vi "Drive Teleop Handler.vi"(10 "Call Context":T1) -> ()   [LabVIEW 2023]
uses:
  swerve/Type Definitions/Data/Robot Velocities.ctl
  <vilib>/Rock Robotics/WPI/DriverStation/WPI_DriverStationDerivedRobotMode.ctl
  Drive/Implementation/Driving Mode.ctl
  <vilib>/Rock Robotics/WPI/Joystick/XBox Buttons Indexer.ctl
  ce51abe2-3967-49ec-91df-d4b8ef358bb3.vi
  20f039dc-a6f5-4e97-88ba-31848a91c715.vi
  2558f998-dd4e-4154-8f44-6f70b21d0474.vi
  fdc21bd4-9215-41b8-8367-bf19dde4ba27.vi
  <vilib>/Rock Robotics/WPI/Utilities/WPI_GetSetVariantRefNum.vi
  <vilib>/Rock Robotics/Network Tables/NT Read Number.vi
  <vilib>/Rock Robotics/Network Tables/NT Read Boolean.vi
  <vilib>/Rock Robotics/Network Tables/NT Write Boolean.vi
  Framework/Robot Global Data.vi
panel:
  in  "Deadband Info":T2={"Deadband"=0.05, "Deadband High"=1.0, "Deadband Low"=0.05}
  in  "Max Velocities":T3={"X Velocity"=15.0, "Y Velocity"=15.0, "Rotational \nVelocity"=270.0}
  in  "Sinusoidal Terms":cluster{"Max Velocity":dbl, "Frequency":dbl}
  in  "Teleop Mode":T4(ring)
  in  "Joystick Inputs":T5(array[cluster])
  in  "Send Inputs":bool
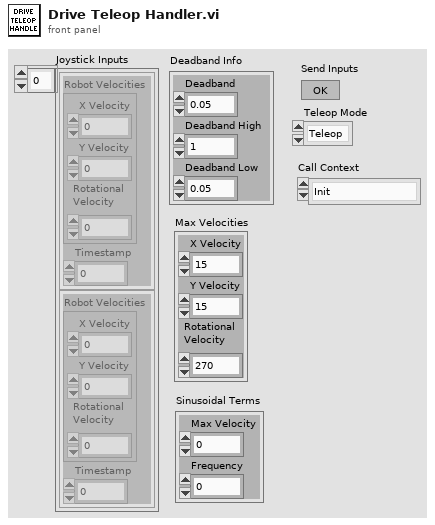
[diagram p1: front panel]
types:
  T1 = typedef "WPI_DriverStationDerivedRobotMode.ctl" = enum16{"Init", "Execute", "Stop"}
  T2 = cluster{"Deadband":dbl, "Deadband High":dbl, "Deadband Low":dbl}
  T3 = typedef "Robot Velocities.ctl" = cluster{"X Velocity":dbl, "Y Velocity":dbl, "Rotational \nVelocity":dbl}
  T4 = enum16{"Teleop", "Simulated Teleop", "Sine Velocity Profiles", "Circle Simulator"}
  T5 = cluster{"Robot Velocities":T3, "Timestamp":dbl}[]
  T6 = typedef "XBox Buttons Indexer.ctl" = enum16{"A", "B", "X", "Y", "Left Bumper", "Right Bumper", "Back", "Start", "Left Joystick", "Right Joystick"}
  T7 = typedef "Driving Mode.ctl" = enum16{"Robot Centric", "Field Centric"}
  T8 = typedef "WPI_JoystickDevRef.ctl" = cluster{"Device":T9}
  T9 = typedef "WPI_JoystickDeviceEnum.ctl" = enum16{"USB 0", "USB 1", "USB 2", "USB 3", "USB 4", "USB 5"}
  T10 = typedef "CTRE_PigeonIMU_DeviceRef.ctl" = cluster{"DeviceStatus":errorcluster, "Device Number":u8, "Type":T11, "Device ID":u32, "Handle":u64, "UsageFrame":u32, "Library Path":path}
  T11 = typedef "CTRE_PigeonIMU_ConnectionType.ctl" = u32
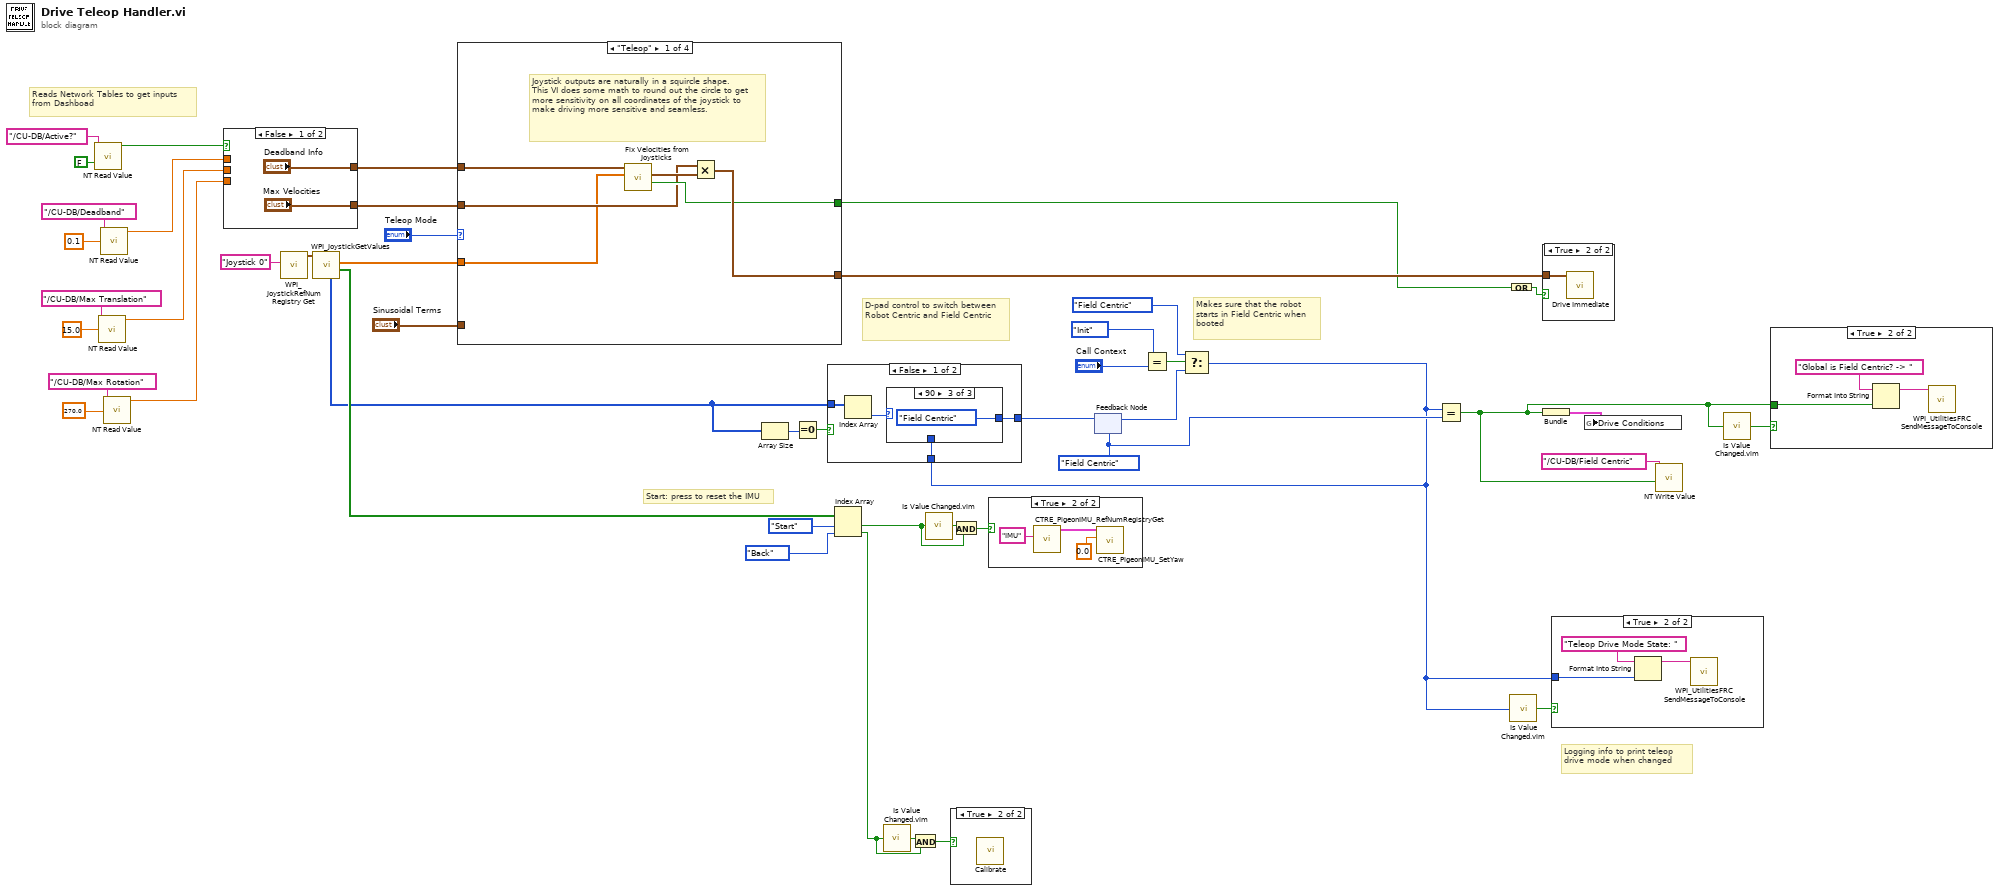
[diagram p0: block diagram]
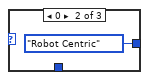
[diagram p7: hidden frame]
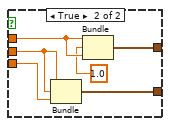
[diagram p9: hidden frame]
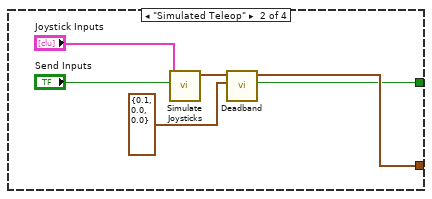
[diagram p10: hidden frame]
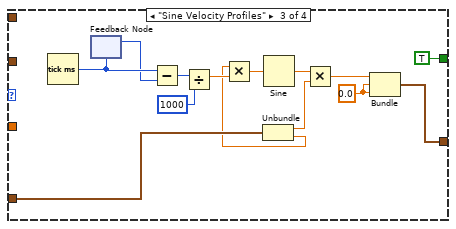
[diagram p11: hidden frame]
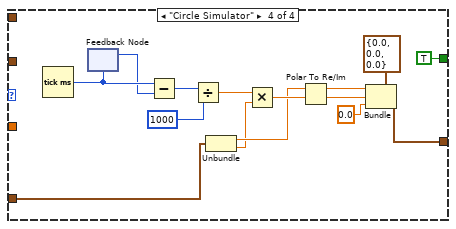
[diagram p12: hidden frame]
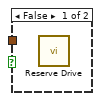
[diagram p13: hidden frame]
diagram:
  w11 = Driving_Mode."Field Centric"
  # "Reads Network Tables to get inputs from Dashboad"
  # "Logging info to print teleop drive mode when changed"
  # "Makes sure that the robot starts in Field Centric when booted"
  # "Start: press to reset the IMU"
  # "D-pad control to switch between Robot Centric and Field Centric"
  n1 = call-poly <vilib>:"NT Read Value.vi"("default value"=FALSE ("Default Value"), "name"="/CU-DB/Active?" ("Name")) -> ("value"=w27:bool)  [unwired: 7 in, 2 out]
  n2 = call-poly <vilib>:"NT Read Value.vi"("default value"=15.0 ("Default Value"), "name"="/CU-DB/Max Translation" ("Name")) -> ("value"=w24:dbl)  [unwired: 7 in, 2 out]
  n3 = call-poly <vilib>:"NT Read Value.vi"("default value"=0.1 ("Default Value"), "name"="/CU-DB/Deadband" ("Name")) -> ("value"=w26:dbl)  [unwired: 7 in, 2 out]
  n4 = call-poly <vilib>:"NT Read Value.vi"("default value"=270.0 ("Default Value"), "name"="/CU-DB/Max Rotation" ("Name")) -> ("value"=w23:dbl)  [unwired: 7 in, 2 out]
  n5 = case shown="False" w27 {
    tunnel: w26 -> [_ w55]
    tunnel: ["Deadband Info" w53] -> w25
    tunnel: w24 -> [_ w52]
    tunnel: w23 -> [_ w51]
    tunnel: ["Max Velocities" w50] -> w22
    frame False {
    }
    frame True {
      n6 = Bundle("value"=w52, "value"=w52, "value"=w51) -> (w50:cluster{"value":dbl, "value":dbl, "value":dbl})  [unwired: 1 in]
      n7 = Bundle("value"=w55, "value"=1.0, "value"=w55) -> (w53:cluster{"value":dbl, "value":dbl, "value":dbl})  [unwired: 1 in]
    }
  }
  n8 = call <vilib>:"WPI_JoystickRefNum Registry Get.vi"("refnum name"="Joystick 0") -> ("JoystickDevRef"=w46:T8)  [unwired: 1 in, 9 out]
  n9 = call <vilib>:"WPI_JoystickGetValues.vi"("JoystickDevRef"=w46) -> ("Buttons"=w43:bool[], "Axes"=w45:dbl[], "POVs"=w18:i16[])  [unwired: 6 in, 2 out]
  n10 = case shown="\"Teleop\"" "Teleop Mode" {
    tunnel: w45 -> [w56 _ _ _]
    tunnel: [w61 w67 w72 w94] -> w38
    tunnel: "Sinusoidal Terms" -> [_ _ w71 w84]
    tunnel: w25 -> [w60 _ _ _]
    tunnel: w22 -> [w57 _ _ _]
    tunnel: [w58 w62 TRUE ("Sending Input?") TRUE ("Sending Input?")] -> w20
    frame "Teleop" {
      # "Joystick outputs are naturally in a squircle shape.\nThis VI does some math to round out the circle to get more sensitivity on all coordinates of the joystick to make driving more sensitive and seamless."
      n11 = call "Fix Velocities from Joysticks.vi"("Axes"=w56, "Deadband"=w60) -> ("Sending Input?"=w58:bool, "Adjusted Robot Velocities"=w59:T3)  [unwired: 8 in]
      n12 = Multiply(x=w57, y=w59) -> (x*y=w61:T3)
    }
    frame "Simulated Teleop" {
      n13 = call "Simulate Joysticks.vi"("Send Inputs"="Send Inputs", "Joystick Inputs"="Joystick Inputs") -> ("Joystick Inputs"=w64:T3)  [unwired: 9 in]
      n14 = call "Deadband.vi"("Deadband Info"=T2 {"Deadband"=0.1, "Deadband High"=0.0, "Deadband Low"=0.0}, "Robot Velocities"=w64) -> ("Sending Input?"=w62:bool, "Adjusted Robot Velocities"=w67:T3)  [unwired: 8 in]
    }
    frame "Sine Velocity Profiles" {
      w80 = 0.0
      n15 = Tick Count (ms)() -> (millisecond timer value=w74:u32)
      n16 = feedback #1(w74) -> (w73:u32)
      n17 = feedback-in #1(w73) -> ()
      n18 = Subtract(x=w74, y=w73) -> (x-y=w78:u32)
      n19 = Divide(x=w78, y=u32 1000) -> (x/y=w76:dbl)
      n20 = Unbundle(w71) -> ("Max Velocity"=w69:dbl, "Frequency"=w70:dbl)
      n21 = Multiply(x=w70, y=w76) -> (x*y=w75:dbl)
      n22 = Sine(x=w75) -> (sin(x)=w79:dbl)
      n23 = Multiply(x=w79, y=w69) -> (x*y=w81:dbl)
      n24 = Bundle(w81, w80, w80) -> (w72:cluster{dbl, dbl, dbl})  [unwired: 1 in]
    }
    frame "Circle Simulator" {
      n25 = Tick Count (ms)() -> (millisecond timer value=w90:u32)
      n26 = feedback #2(w90) -> (w89:u32)
      n27 = feedback-in #2(w89) -> ()
      n28 = Subtract(x=w90, y=w89) -> (x-y=w92:u32)
      n29 = Divide(x=w92, y=u32 1000) -> (x/y=w86:dbl)
      n30 = Unbundle(w84) -> ("Max Velocity"=w87:dbl, "Frequency"=w85:dbl)
      n31 = Multiply(x=w86, y=w85) -> (x*y=w88:dbl)
      n32 = Polar To Re/Im(2:w88, 3:w87) -> (0:w82:dbl, 1:w83:dbl)
      n33 = Bundle(cluster=T3 {"X Velocity"=0.0, "Y Velocity"=0.0, "Rotational \nVelocity"=0.0} ("Robot Velocities (ft/s and deg/s)"), "X Velocity"=w83, "Y Velocity"=w82, "Rotational \nVelocity"=0.0 ("Rotational \nVelocity")) -> (w94:T3)
    }
  }
  n34 = Array Size(array=w18) -> (size(s)=w17:i32)
  n35 = Equal To 0?(x=w17) -> (x = 0?=w16:bool)
  n36 = Index Array(array=w43, index #1=XBox_Buttons_Indexer."Start" ("XBox Buttons"), index #2=XBox_Buttons_Indexer."Back" ("XBox Buttons")) -> (element #1=w40:bool, element #2=w1:bool)
  n37 = call "Is Value Changed.vim"("value"=w1) -> ("changed or first call?"=w5:bool)
  n38 = And(x=w5, y=w1) -> (x .and. y?=w4:bool)
  n39 = call "Is Value Changed.vim"("value"=w40) -> ("changed or first call?"=w41:bool)
  n40 = case shown="True" w4 {
    frame False {
    }
    frame True {
      n41 = call "Calibrate.vi"() -> ()  [unwired: 11 in, 1 out]
    }
  }
  n42 = And(x=w41, y=w40) -> (x .and. y?=w39:bool)
  n43 = case shown="True" w39 {
    frame False {
    }
    frame True {
      n44 = call <vilib>:"CTRE_PigeonIMU_RefNumRegistryGet.vi"("refnum name"="IMU") -> ("PigeonIMUDevRef"=w98:T10)  [unwired: 9 in, 1 out]
      n45 = call <vilib>:"CTRE_PigeonIMU_SetYaw.vi"("Value"=0.0, "PigeonIMUDevRef"=w98) -> ()  [unwired: 8 in, 2 out]
    }
  }
  n46 = feedback #3(w11) -> (w10:T7)
  n47 = Equal?(x=WPI_DriverStationDerivedRobotMode."Init" ("y"), y="Call Context") -> (x = y?=w13:bool)
  n48 = Select(t=Driving_Mode."Field Centric" ("x"), s=w13, f=w10) -> (s? t:f=w7:T7)
  n49 = case shown="False" w16 {
    tunnel: [w102 w107] -> w44
    tunnel: w7 -> [w101 w107]
    tunnel: w18 -> [w100 _]
    frame False {
      n50 = Index Array(array=w100) -> (element=w103:i16)  [unwired: 1 in]
      n51 = case shown="90" w103 {
        tunnel: [w104 Driving_Mode."Robot Centric" Driving_Mode."Field Centric"] -> w102
        tunnel: w101 -> [w104 _ _]
        frame -1, Default {
        }
        frame 0 {
        }
        frame 90 {
        }
      }
    }
    frame True {
    }
  }
  n52 = feedback-in #3(w44) -> ()
  n53 = Equal?(x=w7, y=w11) -> (x = y?=w8:bool)
  n54 = call "Is Value Changed.vim"("value"=w7) -> ("changed or first call?"=w6:bool)
  n55 = Compound Arithmetic op=OR(w20) -> (w21:bool)
  n56 = case shown="True" w21 {
    tunnel: w38 -> [_ w108]
    frame False {
      n57 = call "Reserve Drive.vi"() -> ()  [unwired: 11 in, 1 out]
    }
    frame True {
      n58 = call "Drive Immediate.vi"("Robot Velocities"=w108) -> ()  [unwired: 10 in, 1 out]
    }
  }
  n59 = Bundle(w8) -> (w3:cluster{bool})  [unwired: 1 in]
  n60 = case shown="True" w6 {
    tunnel: w7 -> [_ w109]
    frame False {
    }
    frame True {
      n61 = Format Into String(initial string="Teleop Drive Mode State: ", w109) -> (resulting string=w111:string)  [unwired: 2 in, 1 out]
      n62 = call <vilib>:"WPI_UtilitiesFRC SendMessageToConsole.vi"("Message"=w111) -> ()  [unwired: 14 in, 1 out]
    }
  }
  n63 = global write "Robot Global Data.vi" "Drive Conditions"(w3) -> ()
  n64 = call-poly <vilib>:"NT Write Value.vi"("value"=w8, "name"="/CU-DB/Field Centric") -> ()  [unwired: 9 in, 1 out]
  n65 = call "Is Value Changed.vim"("value"=w8) -> ("changed or first call?"=w9:bool)
  n66 = case shown="True" w9 {
    tunnel: w8 -> [_ w113]
    frame False {
    }
    frame True {
      n67 = Format Into String(initial string="Global is Field Centric? -> ", w113) -> (resulting string=w114:string)  [unwired: 2 in, 1 out]
      n68 = call <vilib>:"WPI_UtilitiesFRC SendMessageToConsole.vi"("Message"=w114) -> ()  [unwired: 14 in, 1 out]
    }
  }
